vi "Digital Input Engine.vi"(5 "Main Engine Q":refnum<queue>, 7 "TCP Enigine Q":refnum<queue>, 8 "error in (no error)":errorcluster, 10 "Engine Name":string, 11 "Varient Data":variant) -> (0 "error out":errorcluster)   [LabVIEW 2024]
doc: "All Rights Reserved © 2023 SyncSols"
uses:
  Controls/Digital Input SM Data Cluster.ctl
  TCP Engine/Controls/TCP Engine I&O  Interupt Cluster.ctl
  Digital Output/Controls/DIO Commad Q Cluster.ctl
  Digital Output/SubVIs/Digital Dynamic Cluster.ctl
  Main Engine/Controls/Main Engine JSON Command State.ctl
  Digital Output/Controls/DIO Configuration cluster.ctl
  Digital Output/Controls/DIO Interface Data.ctl
  Controls/Digital Input SM Cases.ctl
  Main Engine/Controls/Main Engine Engine No.Options.ctl
  Main Engine/Controls/Main Engine Config Confirmation Cluster.ctl
  <vilib>/DAQmx/read.llb/DAQmx Read (Digital 1D Bool NChan 1Samp 1Line).vi
  <vilib>/DAQmx/create/channels.llb/DAQmx Create Channel (DI-Digital Input).vi
  <vilib>/DAQmx/miscellaneous.llb/DAQmx Fill In Error Info.vi
  TCP Engine/TCP Engine.lvlib
panel:
  in  "Data Cluster":T1={"Array"=[], "Boolean"=FALSE, "String"="", "Engine Name"="", "Main Engine Response Q"=refnum, "TCP Engine Response Q"=refnum, "Varient Data"=variant(string ""), "Interupt Q"=refnum, "Command Q"=refnum, "Start Notifier"=refnum, "Stop Notifier"=refnum, "DIO Configuration Cluster"={"Interface"="", "Interface Data"={"Command"="", "SubCmd"="", "Frequency"=0, "Data"=[]}}, "DI Task"="", "Log File Path"=path ""}
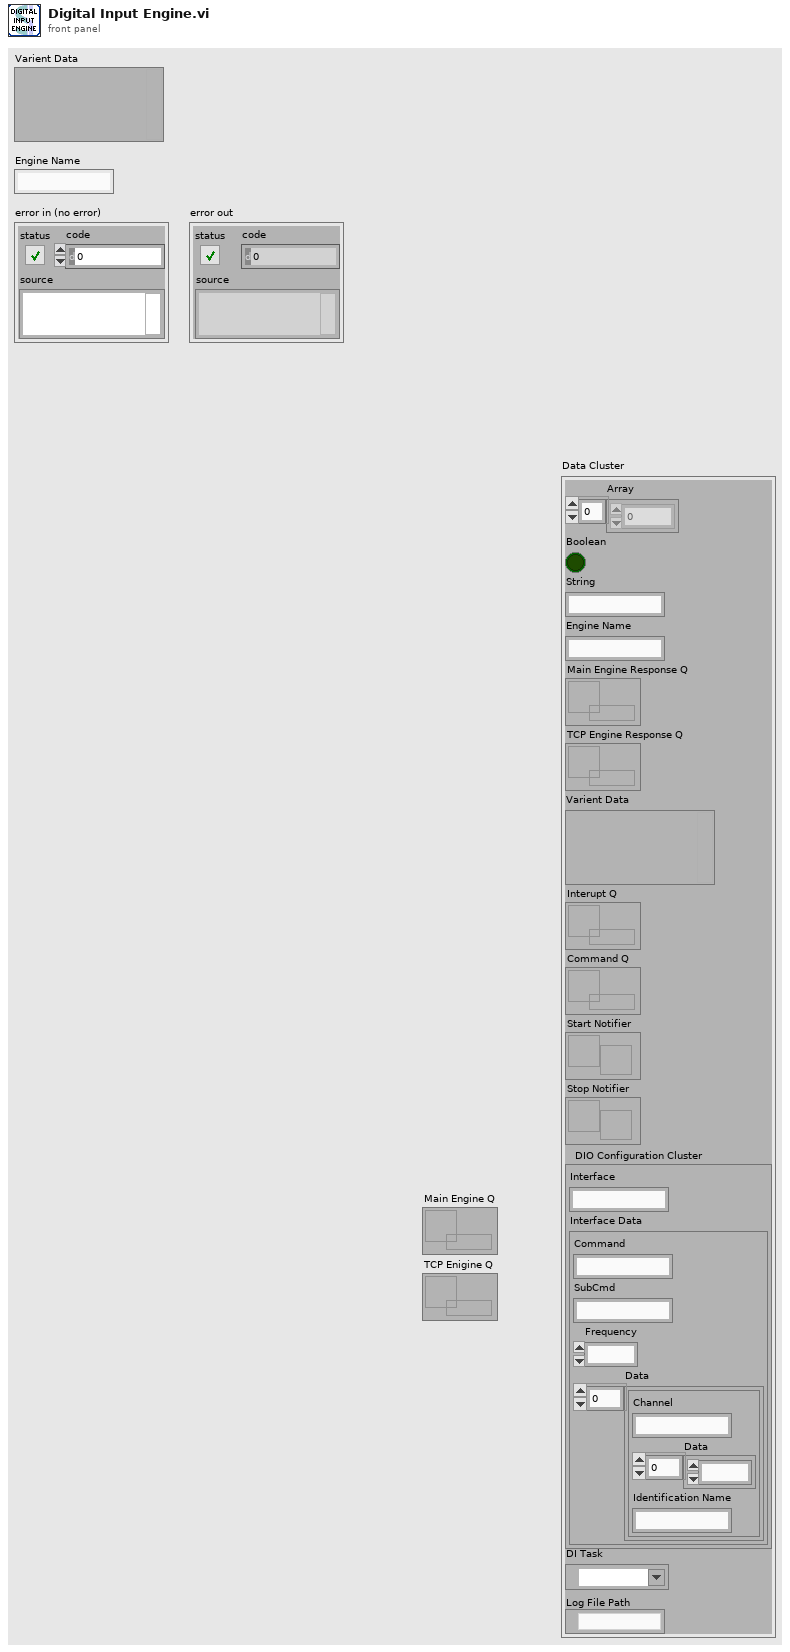
[diagram p1: front panel]
types:
  T1 = typedef "Digital Input SM Data Cluster.ctl" = cluster{"Array":dbl[], "Boolean":bool, "String":string, "Engine Name":string, "Main Engine Response Q":refnum<queue>, "TCP Engine Response Q":refnum<queue>, "Varient Data":variant, "Interupt Q":refnum<queue>, "Command Q":refnum<queue>, "Start Notifier":refnum<notifier>, "Stop Notifier":refnum<notifier>, "DIO Configuration Cluster":T2, "DI Task":refnum<k21>, "Log File Path":path}
  T2 = typedef "DIO Configuration cluster.ctl" = cluster{"Interface":string, "Interface Data":T3}
  T3 = typedef "DIO Interface Data.ctl" = cluster{"Command":string, "SubCmd":string, "Frequency":u16, "Data":T4[]}
  T4 = typedef "Digital Dynamic Cluster.ctl" = cluster{"Channel":string, "Data":u8[], "Identification Name":string}
  T5 = typedef "Digital Input SM Cases.ctl" = enum16{">Poll", ".........State Machine.........", ">Init", ">Error", ">Exit", "..........Digital Input..........", ">JSON to LVDATA", ">Configure", ">Get Command", ">Start", ">Acquire", ">Stop"}
  T6 = typedef "DIO Commad Q Cluster.ctl" = cluster{"Interface":string, "Interface Data":cluster{"Command":string, "SubCmd":string, "Frequency":u16, "Data":T4[]}, "Command State":T7}
  T7 = typedef "Main Engine JSON Command State.ctl" = enum16{"Configure", "Start", "Exit"}
  T8 = typedef "TCP Engine.lvlib/TCP Engine I&O  Interupt Cluster.ctl" = cluster{" Stop":bool, "JSON Variant":variant}
  T9 = typedef "Main Engine Engine No.Options.ctl" = enum16{"Init", "Update", "Response", "Get"}
  T10 = typedef "Main Engine Config Confirmation Cluster.ctl" = cluster{"Command":string, "Interface":string, "Status":string, "Board":string}
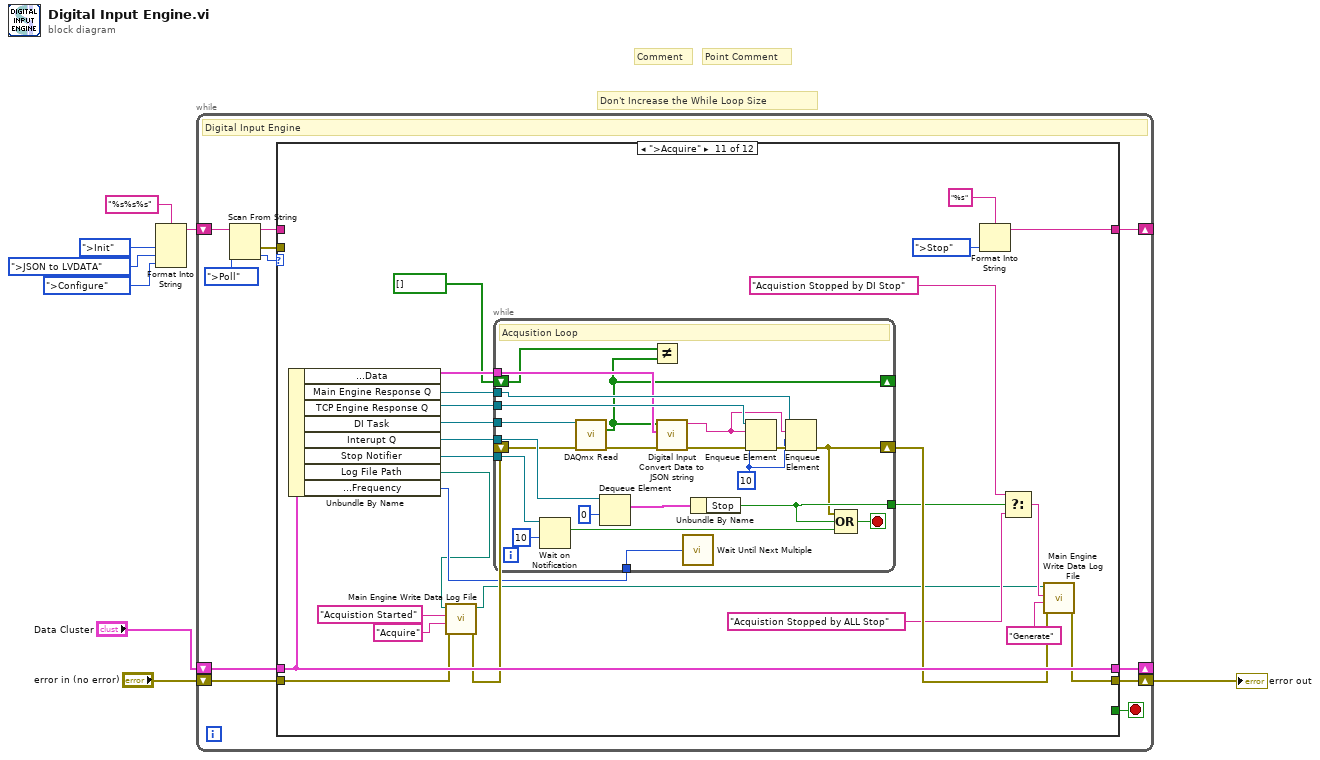
[diagram p0: block diagram]
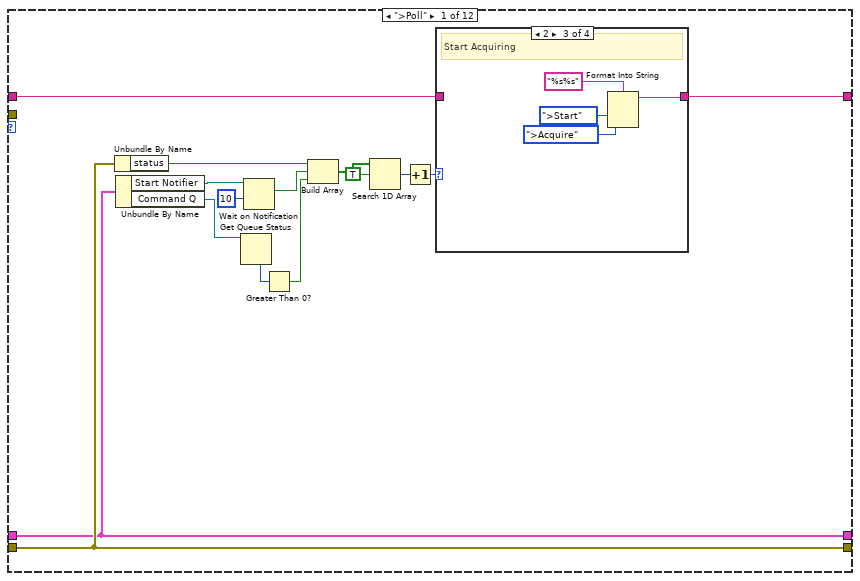
[diagram p2: hidden frame]
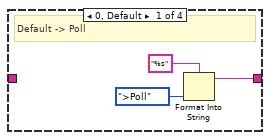
[diagram p3: hidden frame]
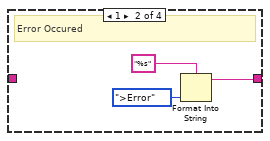
[diagram p4: hidden frame]
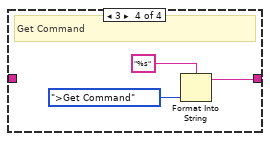
[diagram p5: hidden frame]
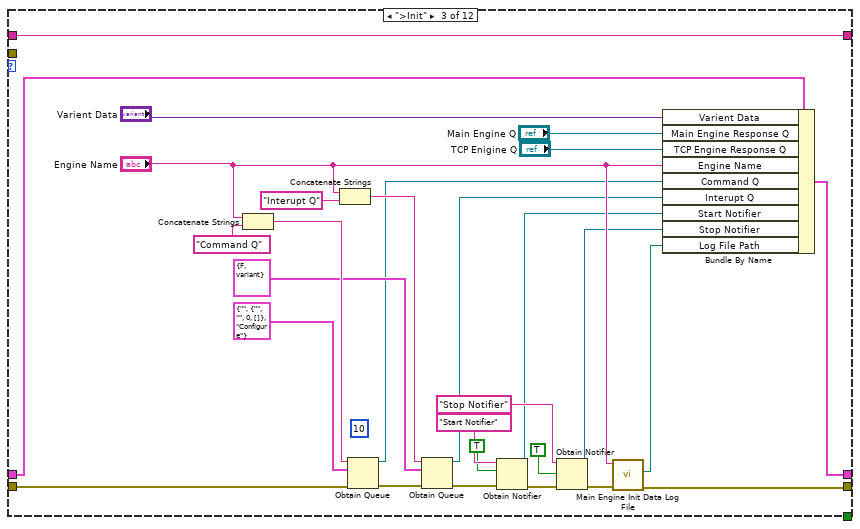
[diagram p7: hidden frame]
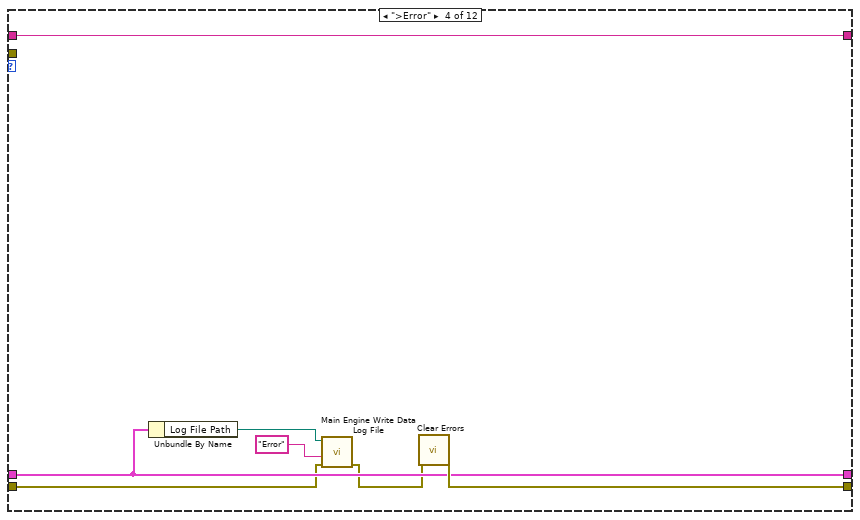
[diagram p8: hidden frame]
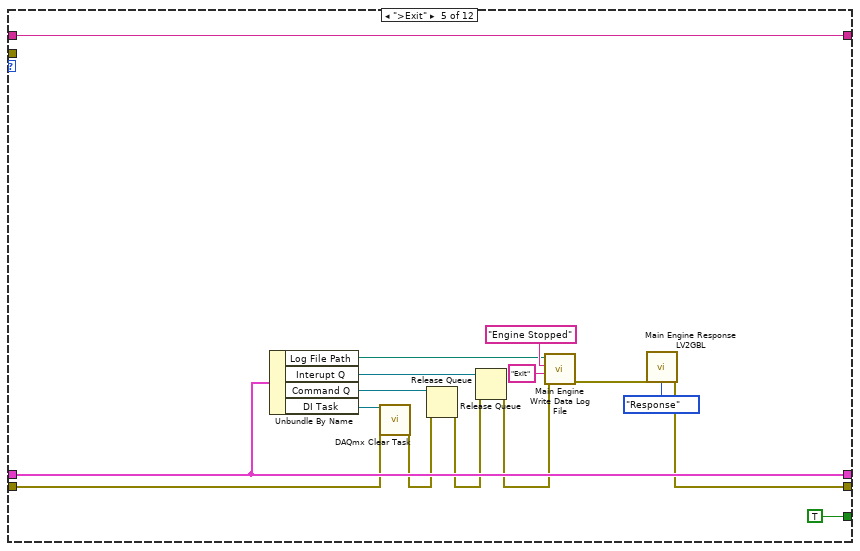
[diagram p9: hidden frame]
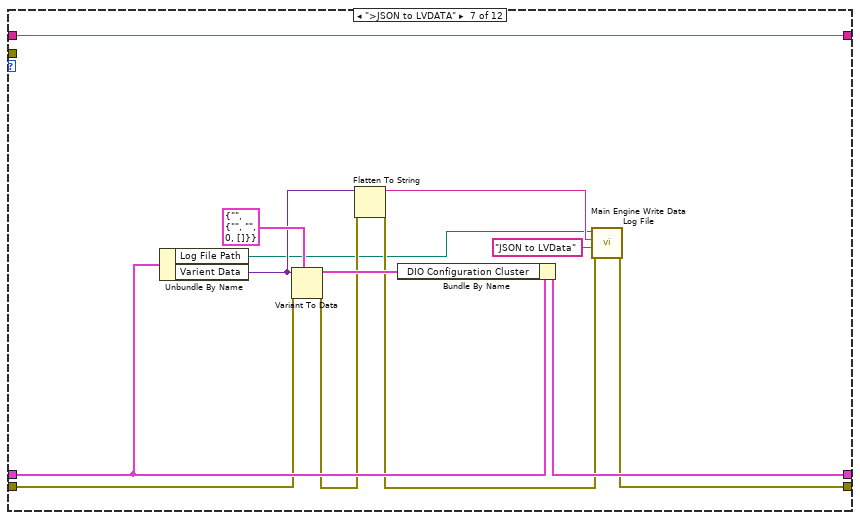
[diagram p11: hidden frame]
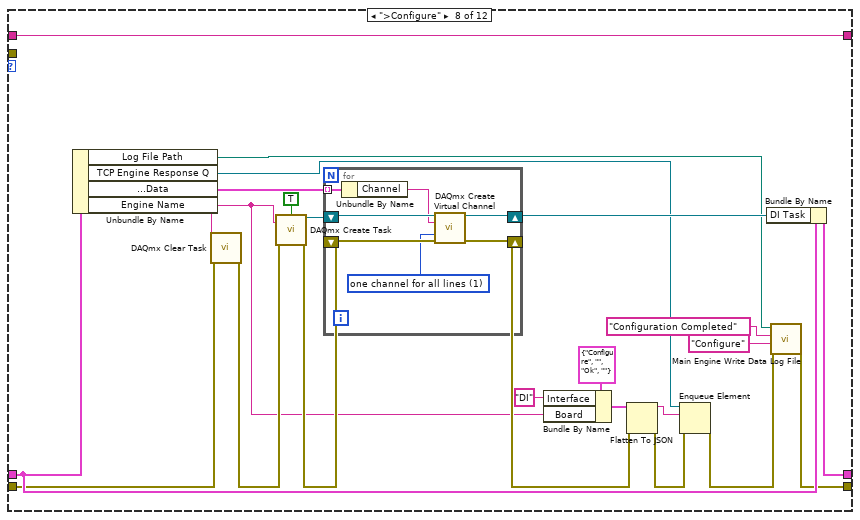
[diagram p12: hidden frame]
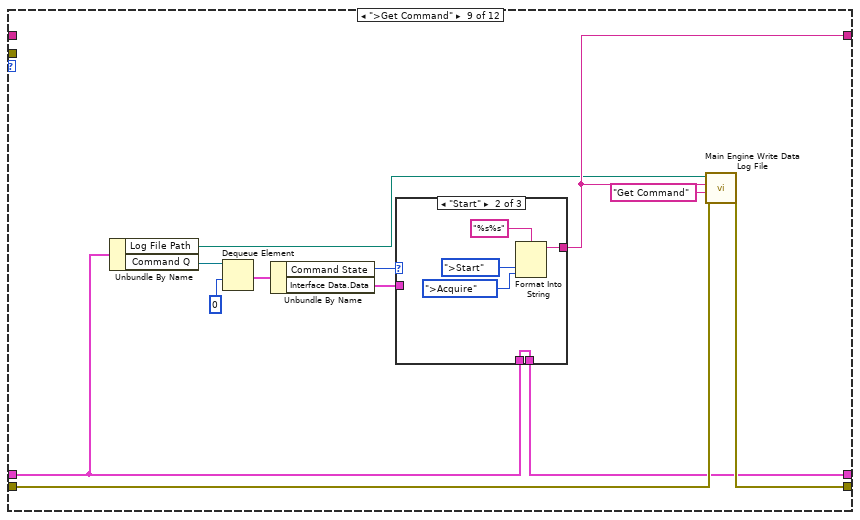
[diagram p13: hidden frame]
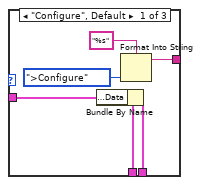
[diagram p14: hidden frame]
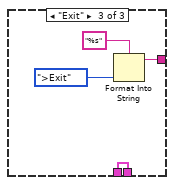
[diagram p15: hidden frame]
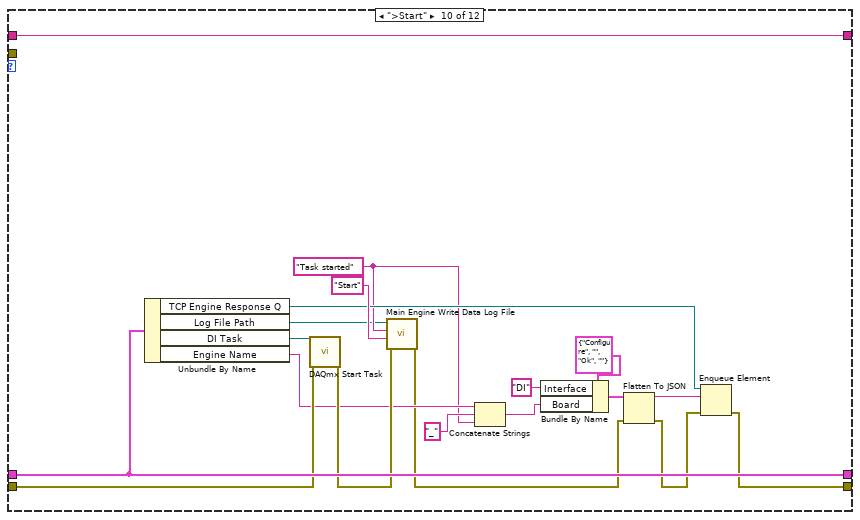
[diagram p16: hidden frame]
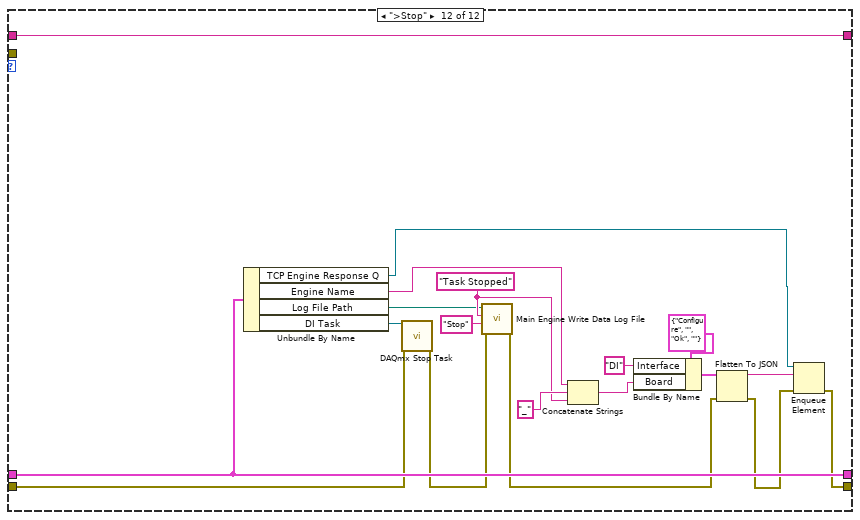
[diagram p17: hidden frame]
diagram:
  # "Don't Increase the While Loop Size"
  # "Point Comment"
  # "Comment"
  n1 = Format Into String(format string="%s%s%s", Digital_Input_SM_Cases.">Init" ("SM Cases Options"), Digital_Input_SM_Cases.">JSON to LVDATA" ("input 2"), Digital_Input_SM_Cases.">Configure" ("input 3")) -> (resulting string=w7:string)  [unwired: 2 in, 1 out]
  n2 = while {
    shift-right: [w14] -> _
    shift-left: w7 -> [w19]
    shift-right: [w12] -> w4
    shift-left: "error in (no error)" -> [w13]
    shift-right: [w10] -> _
    shift-left: "Data Cluster" -> [w9]
    stop <- w11 stop-if-true
    # "Digital Input Engine"
    n3 = Scan From String(input string=w19, default 1=Digital_Input_SM_Cases.">Poll" ("SM Cases Options")) -> (remaining string=w15:string, error out=w17:errorcluster, output 1=w16:T5)  [unwired: 3 in, 1 out]
    n4 = case shown="\">Acquire\"" w16 {
      tunnel: w17 -> [_ _ _ _ _ _ _ _ _ _ _ _]
      tunnel: w15 -> [w34 w50 w78 w85 w101 w104 w117 w140 _ w193 _ w259]
      tunnel: [w33 w50 w78 w85 w101 w104 w117 w140 w151 w193 w211 w259] -> w14
      tunnel: w13 -> [w32 w49 w55 w81 w90 w103 w110 w132 w152 w188 w209 w254]
      tunnel: [w32 w49 w63 w84 w88 w103 w113 w120 w153 w176 w206 w242] -> w12
      tunnel: [_ _ _ _ TRUE _ _ _ _ _ _ _] -> w11
      tunnel: [w22 w48 w62 w82 w95 w102 w115 w134 w150 w190 w218 w256] -> w10
      tunnel: w9 -> [w22 w48 w54 w82 w95 w102 w116 w139 w149 w190 w218 w256]
      frame ">Poll" {
        n5 = Unbundle By Name(w32) -> ("status"=w31:bool)
        n6 = Unbundle By Name(w22) -> ("Start Notifier"=w26:refnum<notifier>, "Command Q"=w24:refnum<queue>)
        n7 = Get Queue Status(queue=w24) -> (# elements in queue=w23:i32)  [unwired: 2 in, 7 out]
        n8 = Wait on Notification(notifier=w26, timeout in ms (-1)=10) -> (notification=w21:bool)  [unwired: 2 in, 3 out]
        n9 = Greater Than 0?(x=w23) -> (x > 0?=w20:bool)
        n10 = Build Array(w31, w21, w20) -> (w30:bool[])
        n11 = Search 1D Array(1D array=w30, element=TRUE) -> (index of element=w28:i32)  [unwired: 1 in]
        n12 = Increment(x=w28) -> (x+1=w27:i32)
        n13 = case shown="2" w27 {
          tunnel: w34 -> [_ _ _ _]
          tunnel: [w35 w38 w42 w45] -> w33
          frame 0, Default {
            # "Default -> Poll"
            n14 = Format Into String(format string="%s", Digital_Input_SM_Cases.">Poll" ("SM Cases Options")) -> (resulting string=w35:string)  [unwired: 2 in, 1 out]
          }
          frame 1 {
            # "Error Occured"
            n15 = Format Into String(format string="%s", Digital_Input_SM_Cases.">Error" ("SM Cases Options")) -> (resulting string=w38:string)  [unwired: 2 in, 1 out]
          }
          frame 2 {
            # "Start Acquiring"
            n16 = Format Into String(format string="%s%s", Digital_Input_SM_Cases.">Start" ("SM Cases Options"), Digital_Input_SM_Cases.">Acquire" ("input 2")) -> (resulting string=w42:string)  [unwired: 2 in, 1 out]
          }
          frame 3 {
            # "Get Command"
            n17 = Format Into String(format string="%s", Digital_Input_SM_Cases.">Get Command" ("SM Cases Options")) -> (resulting string=w45:string)  [unwired: 2 in, 1 out]
          }
        }
      }
      frame ".........State Machine........." {
      }
      frame ">Init" {
        (unwired) 10 ("max queue size (-1, unlimited)")
        n18 = Concatenate Strings("Engine Name", "Command Q" ("string")) -> (w75:string)
        n19 = Concatenate Strings("Engine Name", "Interupt Q" ("string")) -> (w73:string)
        n20 = Obtain Queue(name (unnamed)=w75, element data type=T6 {"Interface"="", "Interface Data"={"Command"="", "SubCmd"="", "Frequency"=0, "Data"=[]}, "Command State"=enum."Configure"} ("DIO Command Q Cluster"), error in (no error)=w55) -> (queue out=w59:refnum<queue>, error out=w77:errorcluster)  [unwired: 2 in, 1 out]
        n21 = Obtain Queue(name (unnamed)=w73, element data type=T8 {" Stop"=FALSE, "JSON Variant"=variant(string "")} ("I/O  Interupt Cluster"), error in (no error)=w77) -> (queue out=w58:refnum<queue>, error out=w65:errorcluster)  [unwired: 2 in, 1 out]
        n22 = Obtain Notifier(name (unnamed)="Start Notifier", notification data type=TRUE, error in (no error)=w65) -> (notifier out=w57:refnum<notifier>, error out=w70:errorcluster)  [unwired: 1 in, 1 out]
        n23 = Obtain Notifier(name (unnamed)="Stop Notifier", notification data type=TRUE, error in (no error)=w70) -> (notifier out=w56:refnum<notifier>, error out=w66:errorcluster)  [unwired: 1 in, 1 out]
        n24 = call "Main Engine Init Data Log File.vi"("error in"=w66, "Engine Name"="Engine Name") -> ("error out"=w63:errorcluster, "Log File Path"=w51:path)  [unwired: 8 in]
        n25 = Bundle By Name(cluster=w54, "Varient Data"="Varient Data", "Main Engine Response Q"="Main Engine Q", "TCP Engine Response Q"="TCP Enigine Q", "Engine Name"="Engine Name", "Command Q"=w59, "Interupt Q"=w58, "Start Notifier"=w57, "Stop Notifier"=w56, "Log File Path"=w51) -> (w62:T1)
      }
      frame ">Error" {
        n26 = Unbundle By Name(w82) -> ("Log File Path"=w79:path)
        n27 = call "Main Engine Write Data Log File.vi"("error in"=w81, "State"="Error" ("Input Data"), "Log file path In"=w79) -> ("error out"=w80:errorcluster)  [unwired: 7 in, 1 out]
        n28 = call <vilib>:"Clear Errors.vi"("error in (no error)"=w80) -> ("error out"=w84:errorcluster)  [unwired: 5 in, 1 out]
      }
      frame ">Exit" {
        n29 = Unbundle By Name(w95) -> ("Log File Path"=w86:path, "Interupt Q"=w98:refnum<queue>, "Command Q"=w99:refnum<queue>, "DI Task"=w89:refnum<k21>)
        n30 = call <vilib>:"DAQmx Clear Task.vi"("task in"=w89, "error in"=w90) -> ("error out"=w91:errorcluster)  [unwired: 13 in]
        n31 = Release Queue(queue=w99, error in (no error)=w91) -> (error out=w94:errorcluster)  [unwired: 1 in, 2 out]
        n32 = Release Queue(queue=w98, error in (no error)=w94) -> (error out=w93:errorcluster)  [unwired: 1 in, 2 out]
        n33 = call "Main Engine Write Data Log File.vi"("error in"=w93, "State"="Exit", "Input Data"="Engine Stopped", "Log file path In"=w86) -> ("error out"=w92:errorcluster)  [unwired: 6 in, 1 out]
        n34 = call "Main Engine Response LV2GBL.vi"("Options"=Main_Engine_Engine_No.Options."Response", "error in"=w92) -> ("error out"=w88:errorcluster)  [unwired: 7 in, 2 out]
      }
      frame "..........Digital Input.........." {
      }
      frame ">JSON to LVDATA" {
        n35 = Unbundle By Name(w116) -> ("Log File Path"=w105:path, "Varient Data"=w109:variant)
        n36 = Variant To Data(error in=w110, type=T2 {"Interface"="", "Interface Data"={"Command"="", "SubCmd"="", "Frequency"=0, "Data"=[]}} ("DIO Configuration Cluster"), Variant=w109) -> (data=w114:T2, error out=w107:errorcluster)
        n37 = Flatten To String(anything=w109, error in (no error)=w107) -> (data string=w108:string, error out=w106:errorcluster)  [unwired: 2 in, 1 out]
        n38 = Bundle By Name(cluster=w116, "DIO Configuration Cluster"=w114) -> (w115:T1)
        n39 = call "Main Engine Write Data Log File.vi"("error in"=w106, "State"="JSON to LVData", "Input Data"=w108, "Log file path In"=w105) -> ("error out"=w113:errorcluster)  [unwired: 6 in, 1 out]
      }
      frame ">Configure" {
        n40 = Unbundle By Name(w139) -> ("Log File Path"=w118:path, "TCP Engine Response Q"=w125:refnum<queue>, "DIO Configuration Cluster.Interface Data.Data"=w135:T4[], "Engine Name"=w124:string)
        n41 = call <vilib>:"DAQmx Clear Task.vi"("task in"=w124, "error in"=w132) -> ("error out"=w138:errorcluster)  [unwired: 13 in]
        n42 = call <vilib>:"DAQmx Create Task.vi"("new task name"=w124, "auto cleanup"=TRUE, "error in"=w138) -> ("task out"=w137:refnum<k21>, "error out"=w136:errorcluster)  [unwired: 11 in]
        n43 = for {
          shift-right: [w143] -> w126
          shift-left: w136 -> [w146]
          shift-right: [w144] -> w133
          shift-left: w137 -> [w147]
          tunnel: w135 -> [w141] mode=indexing
          w145 = 1 items=["one channel for each line", "one channel for all lines"] ("line grouping")
          n44 = Unbundle By Name(w141) -> ("Channel"=w142:string)
          n45 = call-poly <vilib>:"DAQmx Create Virtual Channel.vi"("task in"=w147, "lines"=w142, "line grouping"=w145, "error in"=w146) -> ("task out"=w144:refnum<k21>, "error out"=w143:errorcluster)  [unwired: 10 in]
        }
        n46 = Bundle By Name(cluster=T10 {"Command"="Configure", "Interface"="", "Status"="Ok", "Board"=""}, "Interface"="DI" ("SubCmd"), "Board"=w124) -> (w131:T10)
        n47 = Flatten To JSON(anything=w131, error in (no error)=w126) -> (JSON string=w130:string, 11:w127:errorcluster)  [unwired: 1 in]
        n48 = Enqueue Element(queue=w125, element=w130, error in (no error)=w127) -> (error out=w121:errorcluster)  [unwired: 1 in, 2 out]
        n49 = Bundle By Name(cluster=w139, "DI Task"=w133) -> (w134:T1)
        n50 = call "Main Engine Write Data Log File.vi"("error in"=w121, "State"="Configure", "Input Data"="Configuration Completed", "Log file path In"=w118) -> ("error out"=w120:errorcluster)  [unwired: 6 in, 1 out]
      }
      frame ">Get Command" {
        n51 = Unbundle By Name(w149) -> ("Log File Path"=w148:path, "Command Q"=w159:refnum<queue>)
        n52 = Dequeue Element(queue=w159, timeout in ms (-1)=0) -> (element=w157:T6)  [unwired: 1 in, 3 out]
        n53 = Unbundle By Name(w157) -> ("Command State"=w156:T7, "Interface Data.Data"=w155:T4[])
        n54 = case shown="\"Start\"" w156 {
          tunnel: w149 -> [w165 w170 w174]
          tunnel: w155 -> [w164 _ _]
          tunnel: [w163 w170 w174] -> w150
          tunnel: [w161 w168 w172] -> w151
          frame "Configure", Default {
            n55 = Bundle By Name(cluster=w165, "DIO Configuration Cluster.Interface Data.Data"=w164) -> (w163:T1)
            n56 = Format Into String(format string="%s", Digital_Input_SM_Cases.">Configure" ("input 3")) -> (resulting string=w161:string)  [unwired: 2 in, 1 out]
          }
          frame "Start" {
            n57 = Format Into String(format string="%s%s", Digital_Input_SM_Cases.">Start" ("input 3"), Digital_Input_SM_Cases.">Acquire" ("input 3")) -> (resulting string=w168:string)  [unwired: 2 in, 1 out]
          }
          frame "Exit" {
            n58 = Format Into String(format string="%s", Digital_Input_SM_Cases.">Exit" ("SM Cases Options")) -> (resulting string=w172:string)  [unwired: 2 in, 1 out]
          }
        }
        n59 = call "Main Engine Write Data Log File.vi"("error in"=w152, "State"="Get Command", "Input Data"=w151, "Log file path In"=w148) -> ("error out"=w153:errorcluster)  [unwired: 6 in, 1 out]
      }
      frame ">Start" {
        w182 = "Task started" ("Input Data")
        n60 = Unbundle By Name(w190) -> ("TCP Engine Response Q"=w185:refnum<queue>, "Log File Path"=w175:path, "DI Task"=w192:refnum<k21>, "Engine Name"=w184:string)
        n61 = call <vilib>:"DAQmx Start Task.vi"("task/channels in"=w192, "error in"=w188) -> ("error out"=w189:errorcluster)  [unwired: 12 in, 1 out]
        n62 = call "Main Engine Write Data Log File.vi"("error in"=w189, "State"="Start", "Input Data"=w182, "Log file path In"=w175) -> ("error out"=w178:errorcluster)  [unwired: 6 in, 1 out]
        n63 = Concatenate Strings(w184, "_", w182) -> (w181:string)
        n64 = Bundle By Name(cluster=T10 {"Command"="Configure", "Interface"="", "Status"="Ok", "Board"=""}, "Interface"="DI" ("SubCmd"), "Board"=w181) -> (w179:T10)
        n65 = Flatten To JSON(anything=w179, error in (no error)=w178) -> (JSON string=w187:string, 11:w177:errorcluster)  [unwired: 1 in]
        n66 = Enqueue Element(queue=w185, element=w187, error in (no error)=w177) -> (error out=w176:errorcluster)  [unwired: 1 in, 2 out]
      }
      frame ">Acquire" {
        n67 = Unbundle By Name(w218) -> ("DIO Configuration Cluster.Interface Data.Data"=w198:T4[], "Main Engine Response Q"=w214:refnum<queue>, "TCP Engine Response Q"=w213:refnum<queue>, "DI Task"=w215:refnum<k21>, "Interupt Q"=w217:refnum<queue>, "Stop Notifier"=w216:refnum<notifier>, "Log File Path"=w195:path, "DIO Configuration Cluster.Interface Data.Frequency"=w196:u16)
        n68 = call "Main Engine Write Data Log File.vi"("error in"=w209, "State"="Acquire", "Input Data"="Acquistion Started", "Log file path In"=w195) -> ("error out"=w205:errorcluster, "Log File Path Out"=w194:path)  [unwired: 6 in]
        n69 = while {
          tunnel: w217 -> [w240]
          tunnel: w216 -> [w238]
          tunnel: w215 -> [w233]
          shift-right: [w225] -> w204
          shift-left: w205 -> [w232]
          tunnel: w214 -> [w230]
          tunnel: w213 -> [w231]
          tunnel: [w229] -> w203
          tunnel: w198 -> [w224]
          shift-right: [w223] -> _
          shift-left: bool[] [] ("data") -> [w222]
          tunnel: w196 -> [w221]
          stop <- w235 stop-if-true
          w219 = 10 ("timeout in ms (-1)")
          # "Acqusition Loop"
          n70 = Wait on Notification(notifier=w238, timeout in ms (-1)=10) -> (notification=w234:bool)  [unwired: 2 in, 3 out]
          n71 = call-poly <vilib>:"DAQmx Read.vi"("task/channels in"=w233, "error in"=w232) -> ("data"=w223:bool[], "error out"=w228:errorcluster)  [unwired: 11 in, 1 out]
          n72 = Dequeue Element(queue=w240, timeout in ms (-1)=0) -> (element=w239:T8)  [unwired: 1 in, 3 out]
          n73 = Not Equal?(x=w222, y=w223) -> ()  [unwired: 1 out]
          n74 = call "Digital Input Convert Data to JSON string.vi"("error in"=w228, "DIO Configuration"=w224, "Data In"=w223) -> ("error out"=w226:errorcluster, "JSON String"=w227:string)  [unwired: 7 in]
          n75 = call "Wait Until Next Multiple"("Count(mSec)"=w221) -> ()  [unwired: 1 out]
          n76 = Unbundle By Name(w239) -> ("Stop"=w229:bool)
          n77 = Enqueue Element(queue=w231, element=w227, timeout in ms (-1)=w219, error in (no error)=w226) -> (error out=w220:errorcluster)  [unwired: 2 out]
          n78 = Enqueue Element(queue=w230, element=w227, timeout in ms (-1)=w219, error in (no error)=w220) -> (error out=w225:errorcluster)  [unwired: 2 out]
          n79 = Compound Arithmetic op=OR(w225, w229, w234) -> (w235:bool)
        }
        n80 = Format Into String(format string="%s", Digital_Input_SM_Cases.">Stop" ("input 1")) -> (resulting string=w211:string)  [unwired: 2 in, 1 out]
        n81 = Select(t="Acquistion Stopped by DI Stop" ("State"), s=w203, f="Acquistion Stopped by ALL Stop" ("State")) -> (s? t:f=w199:string)
        n82 = call "Main Engine Write Data Log File.vi"("error in"=w204, "State"="Generate", "Input Data"=w199, "Log file path In"=w194) -> ("error out"=w206:errorcluster)  [unwired: 6 in, 1 out]
      }
      frame ">Stop" {
        w246 = "Task Stopped" ("Input Data")
        n83 = Unbundle By Name(w256) -> ("TCP Engine Response Q"=w247:refnum<queue>, "Engine Name"=w245:string, "Log File Path"=w241:path, "DI Task"=w258:refnum<k21>)
        n84 = call <vilib>:"DAQmx Stop Task.vi"("task/channels in"=w258, "error in"=w254) -> ("error out"=w255:errorcluster)  [unwired: 12 in, 1 out]
        n85 = call "Main Engine Write Data Log File.vi"("error in"=w255, "State"="Stop", "Input Data"=w246, "Log file path In"=w241) -> ("error out"=w244:errorcluster)  [unwired: 6 in, 1 out]
        n86 = Concatenate Strings(w245, "_", w246) -> (w250:string)
        n87 = Bundle By Name(cluster=T10 {"Command"="Configure", "Interface"="", "Status"="Ok", "Board"=""}, "Interface"="DI" ("SubCmd"), "Board"=w250) -> (w248:T10)
        n88 = Flatten To JSON(anything=w248, error in (no error)=w244) -> (JSON string=w253:string, 11:w243:errorcluster)  [unwired: 1 in]
        n89 = Enqueue Element(queue=w247, element=w253, error in (no error)=w243) -> (error out=w242:errorcluster)  [unwired: 1 in, 2 out]
      }
    }
  }
  "error out" <- w4
